vi "GenerationConfig.vi"(8 "error in (no error)":errorcluster, 11 "GenerationConfig":T1={"ExternalAtt"=0.0, "Freq"=5180000000.0, "RxPwr"=-40.0, "PortName"=6, "PacketNumber"=100, "WaveformName(WithType)"="ac80mcs9.tdms"} {"RxPwr" format="%#_13g"; "Freq" format="%#_13g"; "ExternalAtt" format="%#_13g"}) -> (0 "error out":errorcluster, 3 "GenerationConfigCMD":string[](array[string])=["SOUR:RFSG:GPRF:EATTenuation 0", "SOUR:RFSG:GPRF:FREQ 5180000000", "SOUR:RFSG:GPRF:LEVel -40", "SOUR:RFSG:GPRF:PORT 'Port0'", "SOUR:RFSG:GPRF:ARB:CYCL 0", "SOUR:RFSG:GPRF:ARB:REP FINITE", "SOUR:RFSG:GPRF:ARB:WAV ''", "SOUR:RFSG:GPRF:MODE  ARB", "*OPC?"])   [LabVIEW 2015]
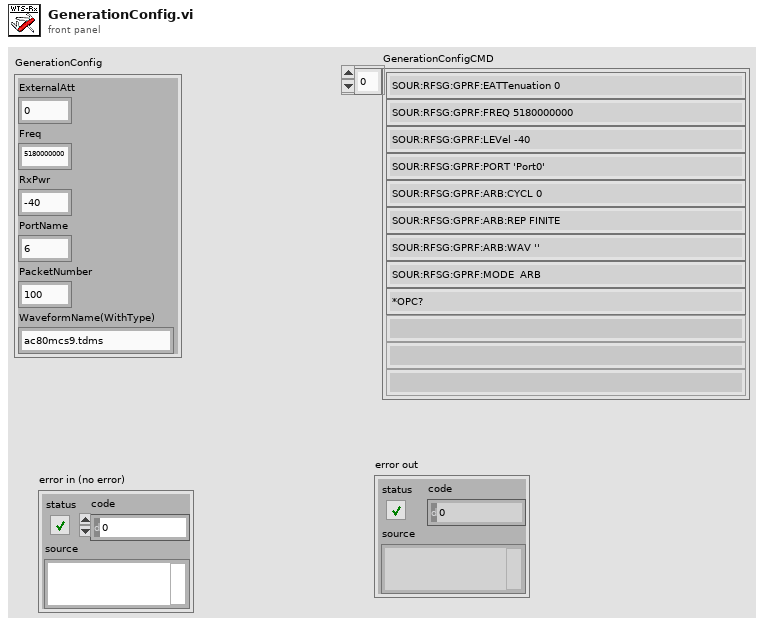
[diagram p1: front panel]
types:
  T1 = cluster{"ExternalAtt":dbl, "Freq":dbl, "RxPwr":dbl, "PortName":i32, "PacketNumber":i32, "WaveformName(WithType)":string}
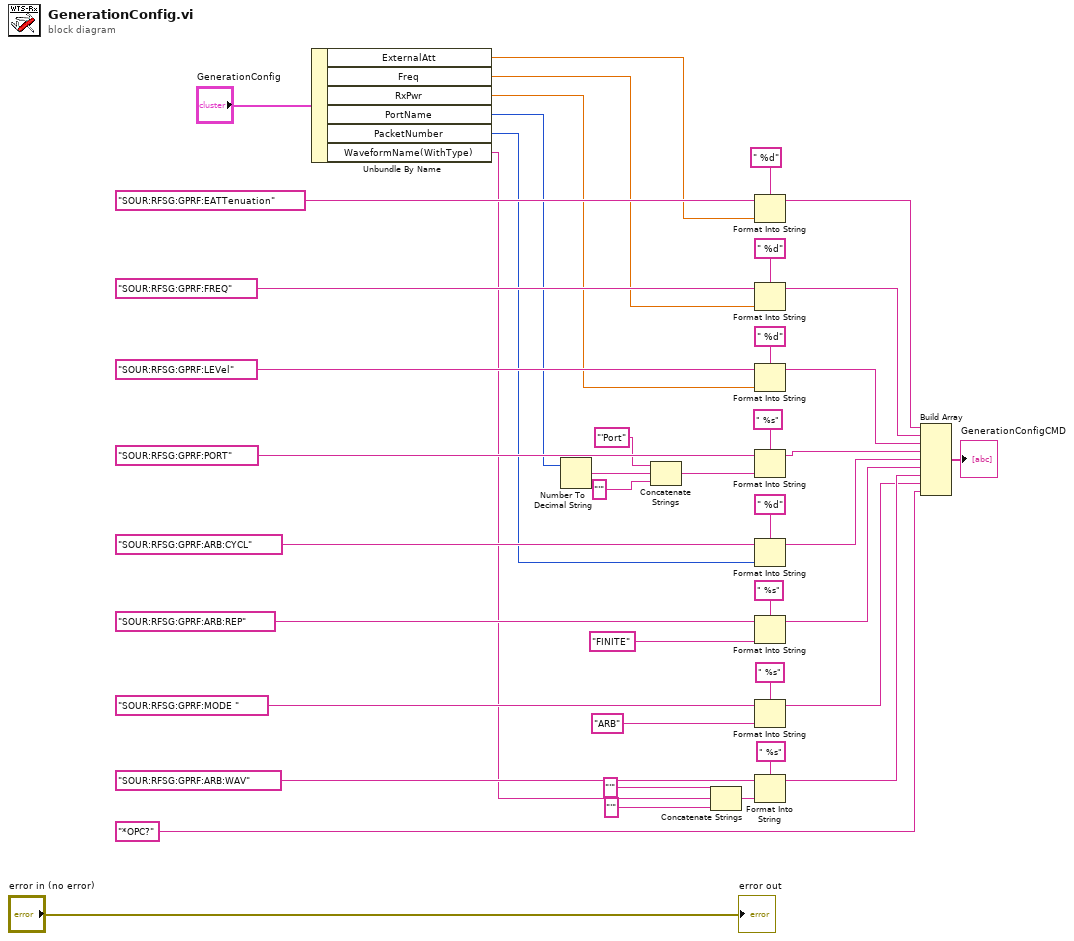
[diagram p0: block diagram]
diagram:
  n1 = Unbundle By Name("GenerationConfig") -> ("ExternalAtt"=w7:dbl, "Freq"=w6:dbl, "RxPwr"=w5:dbl, "PortName"=w4:i32, "PacketNumber"=w3:i32, "WaveformName(WithType)"=w2:string)
  n2 = Number To Decimal String(number=w4) -> (decimal integer string=w26:string)  [unwired: 1 in]
  n3 = Concatenate Strings("'Port", w26, "'" ("string")) -> (w25:string)
  n4 = Concatenate Strings("'", w2, "'" ("string")) -> (w22:string)
  n5 = Format Into String(format string=" %d", initial string="SOUR:RFSG:GPRF:EATTenuation", w7) -> (resulting string=w21:string)  [unwired: 1 in, 1 out]
  n6 = Format Into String(format string=" %d", initial string="SOUR:RFSG:GPRF:FREQ", w6) -> (resulting string=w20:string)  [unwired: 1 in, 1 out]
  n7 = Format Into String(format string=" %d", initial string="SOUR:RFSG:GPRF:LEVel", w5) -> (resulting string=w19:string)  [unwired: 1 in, 1 out]
  n8 = Format Into String(format string=" %s", initial string="SOUR:RFSG:GPRF:PORT", w25) -> (resulting string=w18:string)  [unwired: 1 in, 1 out]
  n9 = Format Into String(format string=" %d", initial string="SOUR:RFSG:GPRF:ARB:CYCL", w3) -> (resulting string=w17:string)  [unwired: 1 in, 1 out]
  n10 = Format Into String(format string=" %s", initial string="SOUR:RFSG:GPRF:ARB:REP", "FINITE" ("input 1")) -> (resulting string=w16:string)  [unwired: 1 in, 1 out]
  n11 = Format Into String(format string=" %s", initial string="SOUR:RFSG:GPRF:MODE ", "ARB" ("input 1")) -> (resulting string=w14:string)  [unwired: 1 in, 1 out]
  n12 = Format Into String(format string=" %s", initial string="SOUR:RFSG:GPRF:ARB:WAV", w22) -> (resulting string=w15:string)  [unwired: 1 in, 1 out]
  n13 = Build Array(w21, w20, w19, w18, w17, w16, w15, w14, "*OPC?") -> (→"GenerationConfigCMD":string[])
  "error out" <- "error in (no error)"
